vi "PickActiveTeam.vi"(0 "Robots":refnum<class "Robot.lvclass">[](array[class]), 2 "AllyTeamArray":T1[](array[typedef]), 4 "Team":T1, 5 "error in (no error)":errorcluster) -> (14 "Robots out":refnum<class "Robot.lvclass">[](array[class]), 19 "error out":errorcluster)   [LabVIEW 2023, in "Ally.lvclass"]
uses:
  Ally.lvclass
  Controls/AllyTeam.ctl
  Robot_class/Robot.lvclass
  Robot_class/Robot.lvclass/Robot.ctl
  Robot_class/Read id.vi
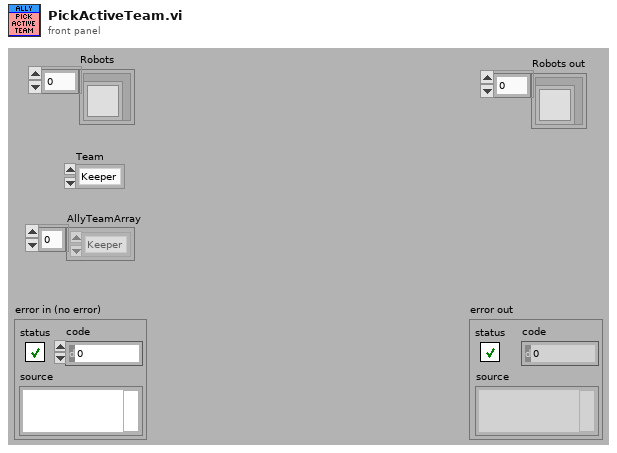
[diagram p1: front panel]
types:
  T1 = typedef "AllyTeam.ctl" = enum16{"Keeper", "Defender", "Attacker"}
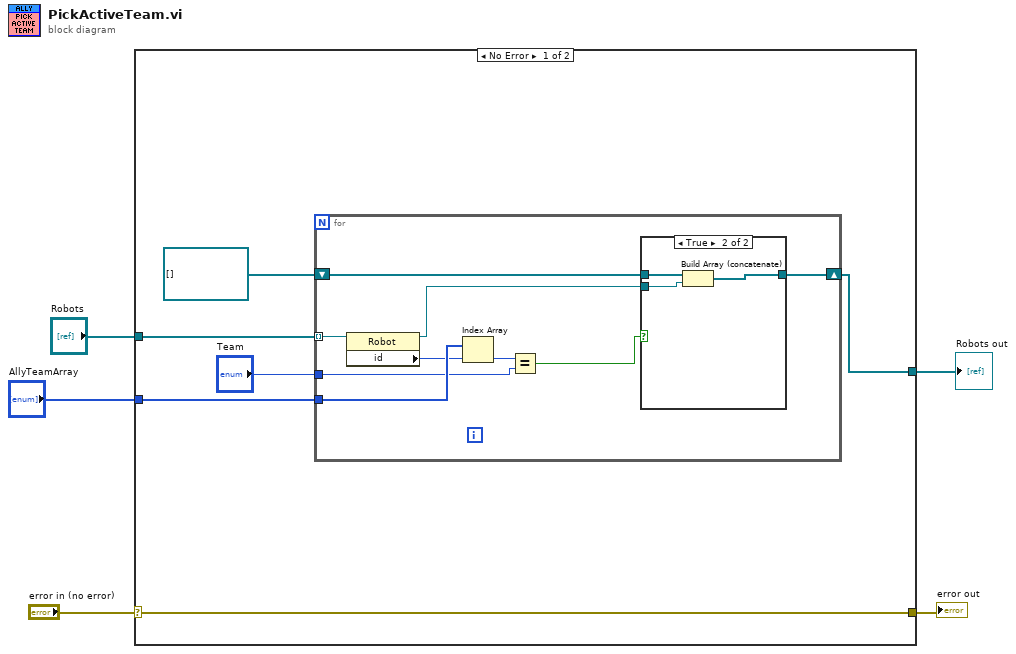
[diagram p0: block diagram]
diagram:
  n1 = case shown="No Error" "error in (no error)" {
    selector: "error in (no error)" -> [w11 w26]
    tunnel: [w11 w26] -> w4
    tunnel: [w9 w25] -> w3
    tunnel: "Robots" -> [w8 w25]
    tunnel: "AllyTeamArray" -> [w7 _]
    frame No Error {
      n2 = for {
        shift-right: [w13] -> w9
        shift-left: refnum<class "Robot.lvclass">[] [] ("Array") -> [w20]
        tunnel: w8 -> [w19] mode=indexing
        tunnel: w7 -> [w18]
        tunnel: "Team" -> [w16]
        n3 = property class="Robot"(reference=w19) -> (reference out=w14:refnum<class "Robot.lvclass">, "id"=w15:i32)  [unwired: 1 in, 1 out]
        n4 = Index Array(array=w18, index=w15) -> (element=w17:T1)
        n5 = Equal?(x=w17, y=w16) -> (x = y?=w12:bool)
        n6 = case shown="True" w12 {
          tunnel: w20 -> [w21 w24]
          tunnel: [w21 w23] -> w13
          tunnel: w14 -> [_ w22]
          frame False {
          }
          frame True {
            n7 = Build Array (concatenate)(w24, w22) -> (w23:refnum<class "Robot.lvclass">[])
          }
        }
      }
    }
    frame Error {
    }
  }
  "error out" <- w4
  "Robots out" <- w3
